vi "Set micron_MessageReply.vi"(7 "Complete Call (T)":bool=TRUE, 8 "error in (no error)":errorcluster, 10 "package_templatemessage":T1, 11 "gRPCid":T3) -> (0 "error out":errorcluster)   [LabVIEW 2019, in "Micron_server.lvlib"]
uses:
  Micron_server.lvlib
  <vilib>/gRPC/LabVIEW gRPC Library/Shared/grpcId.ctl
  micron_MessageReply.ctl
  micron_MessageReply_Status.ctl
  micron_MessageReply_Flat.ctl
  micron_MessageReply_Status_Flat.ctl
  dcc74a39-081a-4bdd-860b-8ed792803c96.vi
  RichToFlatmicron_MessageReply_Status.vi
  <vilib>/gRPC/LabVIEW gRPC Library/Shared/TranslateGrpcError.vi
  <vilib>/gRPC/LabVIEW gRPC Library/Server API/Server/Get Server DLL Path.vi
  <vilib>/Utility/error.llb/Error Cluster From Error Code.vi
  <vilib>/gRPC/LabVIEW gRPC Library/grpc-lvsupport-release.lvlib
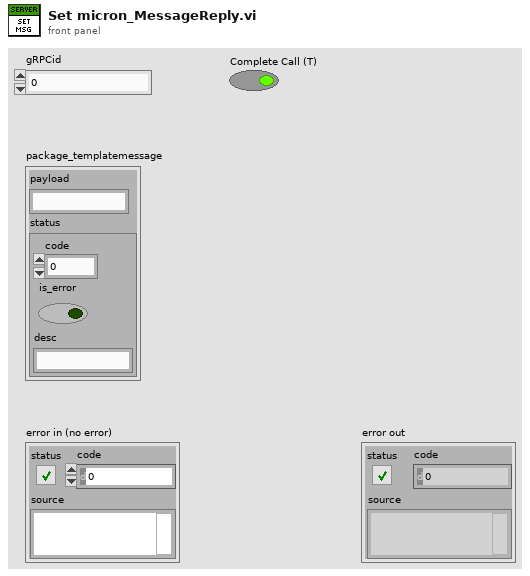
[diagram p1: front panel]
types:
  T1 = typedef "Micron_server.lvlib/micron_MessageReply.ctl" = cluster{"payload":string, "status":T2}
  T2 = typedef "Micron_server.lvlib/micron_MessageReply_Status.ctl" = cluster{"code":i32, "is_error":bool, "desc":string}
  T3 = typedef "grpc-lvsupport-release.lvlib/grpcId.ctl" = u64
  T4 = typedef "Micron_server.lvlib/micron_MessageReply_Flat.ctl" = cluster{"payload":string, "status":T5}
  T5 = typedef "Micron_server.lvlib/micron_MessageReply_Status_Flat.ctl" = cluster{"code":i32, "is_error":bool, "desc":string}
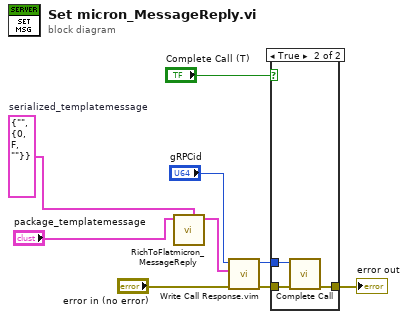
[diagram p0: block diagram]
diagram:
  w2 = T4 {"payload"="", "status"={"code"=0, "is_error"=FALSE, "desc"=""}}  # serialized_templatemessage
  n1 = call "RichToFlatmicron_MessageReply.vi"("OutputClusterType"=w2, "InputCluster"="package_templatemessage") -> ("OutputCluster"=w1:T4)  [unwired: 9 in]
  n2 = call "Write Call Response.vim"("error in"="error in (no error)", "Response Data"=w1, "gRPCid in"="gRPCid") -> ("error out"=w6:errorcluster, "gRPCid out"=w7:T3)  [unwired: 7 in]
  n3 = case shown="True" "Complete Call (T)" {
    tunnel: [w10 w13] -> w9
    tunnel: w7 -> [_ w12]
    tunnel: w6 -> [w10 w11]
    frame False {
    }
    frame True {
      n4 = call <vilib>:"Complete Call.vi"("gRPCid"=w12, "error in"=w11) -> ("error out"=w13:errorcluster)  [unwired: 8 in]
    }
  }
  "error out" <- w9
